vi "write eight integers to csv line and file.vi"(0 "Path":path, 1 "item 3":u32, 2 "item 2":u32, 3 "item 1":u32, 5 "item 4":u32, 7 "item 5":u32, 9 "item 6":u32, 11 "error in (no error)":errorcluster, 12 "item 7":u32, 13 "item 8":u32) -> (4 "concatenated string":string, 15 "error out":errorcluster)   [LabVIEW 2013]
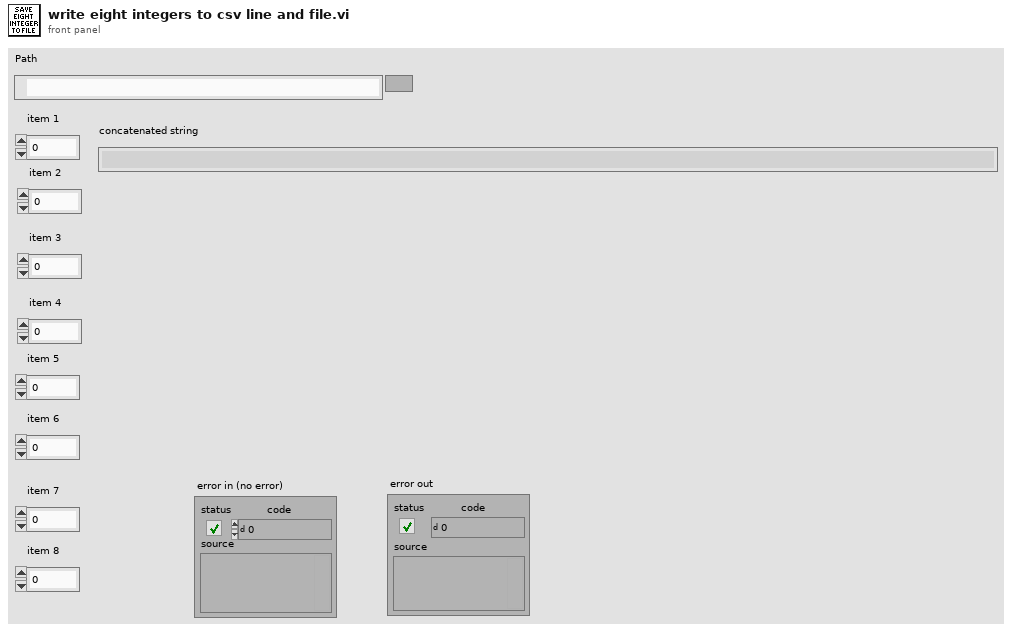
[diagram p1: front panel]
types:
  T1 = enum16{"open", "replace", "create", "open or create", "replace or create", "replace or create with confirmation"}
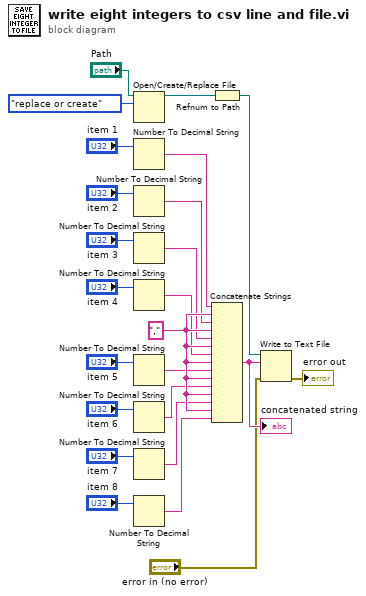
[diagram p0: block diagram]
diagram:
  w21 = "," ("element")
  n1 = Open/Create/Replace File(file path (use dialog)="Path", operation (0:open)=T1."replace or create") -> (refnum out=w24:refnum<file>)  [unwired: 4 in, 2 out]
  n2 = Number To Decimal String(number="item 1") -> (decimal integer string=w12:string)  [unwired: 1 in]
  n3 = Number To Decimal String(number="item 2") -> (decimal integer string=w11:string)  [unwired: 1 in]
  n4 = Number To Decimal String(number="item 3") -> (decimal integer string=w10:string)  [unwired: 1 in]
  n5 = Number To Decimal String(number="item 4") -> (decimal integer string=w9:string)  [unwired: 1 in]
  n6 = Number To Decimal String(number="item 5") -> (decimal integer string=w8:string)  [unwired: 1 in]
  n7 = Number To Decimal String(number="item 6") -> (decimal integer string=w7:string)  [unwired: 1 in]
  n8 = Number To Decimal String(number="item 7") -> (decimal integer string=w6:string)  [unwired: 1 in]
  n9 = Number To Decimal String(number="item 8") -> (decimal integer string=w5:string)  [unwired: 1 in]
  n10 = Refnum to Path(1:w24) -> (0:w4:path)
  n11 = Concatenate Strings(w12, w21, w11, w21, w10, w21, w9, w21, w8, w21, w7, w21, w6, w21, w5) -> (w3:string)
  "concatenated string" <- w3
  n12 = Write to Text File(file (use dialog)=w4, text=w3, error in="error in (no error)") -> (error out=→"error out":errorcluster)  [unwired: 1 in, 2 out]
